vi "PH_BackreflectionMeas.constructor.vi"(0 "name":string, 2 "data in":string, 5 "error in(no error)":errorcluster) -> (14 "i ref out":refnum<vi>, 16 "data out":string, 19 "error out":errorcluster)   [LabVIEW 2014, in "PH_BackreflectionMeas.lvlib"]
doc: "This is the constructor of a class.\n\nLicense Agreement for this software:\n\nCopyright (C)\nGesellschaft für Schwerionenforschung, GSI\nPlanckstr. 1\n64291 Darmstadt\nGermany\n\nContact: D.Beck@gsi.de \n\nThis program is free software; you can redistribute it and/or modify it under the terms of the \nGNU General Public License as published by the Free Software Foundation; either version 2 of \nthe license, or (at your option) any later version.\n\nThis program is distributed in the hope that it will be useful, but WITHOUT ANY WARRANTY; \nwithout even the implied warranty of MERCHANTABILITY or FITNESS FOR A PARTICULAR PURPOSE. See the GNU General License for more details (http://www.gnu.org).\n\nGesellschaft für Schwerionenforschung, GSI\nPlanckstr. 1, 64291 Darmstadt, Germany\nFor all questions and ideas contact: M.Richter@gsi.de, H.Brand@gsi.de or D.Beck@gsi.de.\nLast update: 16-JUN-2004"
uses:
  PH_BackreflectionMeas.lvlib
  CS_Core/CSSystem/CSSystemLib/CSSystemLib.lvlib
  PH_Devices/PH_TKTDS-30xx/PH_TKTDS-30xx.lvlib
  PH_Basics/PH_Class/PH_Class.lvlib
  PH_Basics/PH_StatusHandler/PH_StatusHandler.lvlib
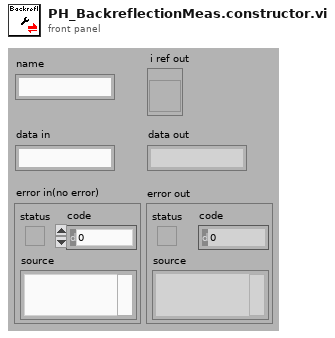
[diagram p1: front panel]
types:
  T1 = enum16{"SetAttribute", "GetAttribute", "CreateAttribute", "DestroyAttribute", "DestroyAllAtributes"}
  T2 = typedef "PH_BackreflectionMeas.lvlib/PH_BackreflectionMeas.i attribute.ctl" = cluster{"GUI Refs":cluster{"Get Data":refnum<vi>, "BR State":refnum<vi>, "Reset warning":refnum<vi>, "Low Energy Graph":refnum<vi>}, "Status":cluster{"Reset Warning":bool}, "Default Low Energy Chan Settings":T3, "Default High Energy Chan Settings":T3, "Default Trigger Settings":T4, "Default Acqu Settings":T5, "Limit [V]":dbl}
  T3 = typedef "PH_TKTDS-30xx.lvlib/PH_TKTDS-30xx.Channel Config.ctl" = cluster{"Channel Name":string, "Input Impedance":string, "Max Input Frequency":string, "Vertical Coupling":i32, "Channel Enabled":bool, "Probe Attenuation":dbl, "Vertical Range":dbl, "Vertical Offset":dbl}
  T4 = typedef "PH_TKTDS-30xx.lvlib/PH_TKTDS-30xx.Trigger Config.ctl" = cluster{"Source":string, "Slope":i32, "Level [V]":dbl}
  T5 = typedef "PH_TKTDS-30xx.lvlib/PH_TKTDS-30xx.Acquisition Config.ctl" = cluster{"Time base":dbl, "Record Length":u16, "Start Time":dbl, "Type":i32, "Continuous":bool}
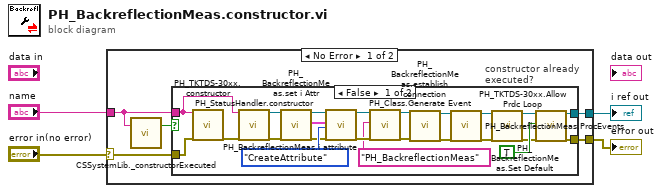
[diagram p0: block diagram]
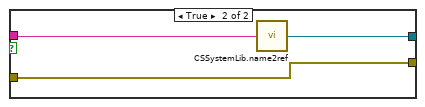
[diagram p2: hidden frame]
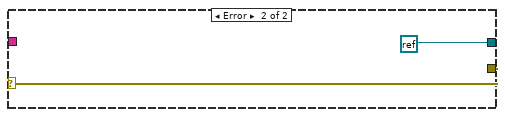
[diagram p3: hidden frame]
diagram:
  n1 = case shown="No Error" "error in(no error)" {
    selector: "error in(no error)" -> [w7 w36]
    tunnel: "name" -> [w5 _]
    tunnel: [w9 refnum<k0> refnum] -> w3
    tunnel: [w8 w36] -> w2
    frame No Error {
      n2 = call "CSSystemLib._constructorExecuted.vi"("name"=w5) -> ("constructor executed?"=w6:bool)  [unwired: 18 in]
      n3 = case "constructor already executed?" shown="False" w6 {
        tunnel: [w27 w34] -> w9
        tunnel: [w26 w33] -> w8
        tunnel: w7 -> [w17 w33]
        tunnel: w5 -> [w10 w35]
        frame False {
          n4 = call "PH_TKTDS-30xx.constructor.vi"("name"=w10, "error in(no error)"=w17) -> ("error out"=w12:errorcluster)  [unwired: 15 in, 2 out]
          n5 = call "PH_StatusHandler.constructor.vi"("name"=w10, "error in(no error)"=w12) -> ("i ref out"=w13:refnum<vi>, "error out"=w11:errorcluster)  [unwired: 15 in, 1 out]
          n6 = call "PH_BackreflectionMeas.set i Attr.vi"("i ref in"=w13, "error in (no error)"=w11) -> ("i ref out"=w15:refnum<vi>, "i Attributes"=w16:T2, "error out"=w14:errorcluster)  [unwired: 15 in]
          n7 = call "PH_BackreflectionMeas.i attribute.vi"("VI Refnum"=w15, "CLASS.i attribute"=w16, "Action"=T1."CreateAttribute", "error in (no error)"=w14) -> ("VI Refnum out"=w22:refnum<vi>, "error out"=w21:errorcluster)  [unwired: 13 in, 1 out]
          n8 = call "PH_Class.Generate Event.vi"("i ref in"=w22, "Class"="PH_BackreflectionMeas", "error in (no error)"=w21) -> ("i ref out"=w20:refnum<vi>, "error out"=w19:errorcluster)  [unwired: 15 in]
          n9 = call "PH_BackreflectionMeas.establish connection.vi"("i ref in"=w20, "error in"=w19) -> ("i ref out"=w30:refnum<vi>, "error out"=w32:errorcluster)  [unwired: 16 in]
          n10 = call "PH_BackreflectionMeas.ProcEvents.vi"("i ref in"=w30, "error in"=w32) -> ("i ref out"=w29:refnum<vi>, "error out"=w31:errorcluster)  [unwired: 16 in]
          n11 = call "PH_BackreflectionMeas.Set Default.vi"("i ref in"=w29, "error in"=w31) -> ("i ref out"=w24:refnum<vi>, "error out"=w23:errorcluster)  [unwired: 16 in]
          n12 = call "PH_TKTDS-30xx.Allow Prdc Loop.vi"("i ref in"=w24, "Allow Prdc Loop?"=TRUE ("constructor finished?"), "error in"=w23) -> ("i ref out"=w27:refnum<vi>, "error out"=w26:errorcluster)  [unwired: 15 in]
        }
        frame True {
          n13 = call "CSSystemLib.name2ref.vi"("name"=w35) -> ("obj refnum"=w34:refnum<vi>)
        }
      }
    }
    frame Error {
    }
  }
  "i ref out" <- w3
  "error out" <- w2
